vi "ODSS_Gen_Script.vi"(7 "Path":path, 8 "error in (no error)":errorcluster, 10 "Time":i32[](array[numeric]), 11 "Main Str":string) -> (0 "error out":errorcluster)   [LabVIEW 2010]
doc: "This Vi implements the routine for writing the simulation script for the next simulation step in OpenDSS.\n\nCreated by Davis Montenegro\n29-06-2017"
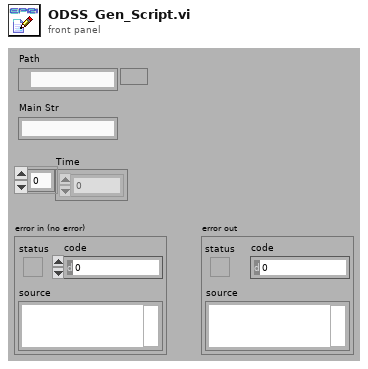
[diagram p1: front panel]
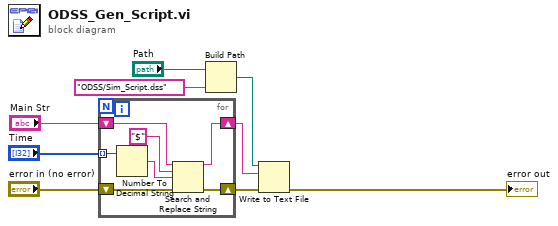
[diagram p0: block diagram]
diagram:
  n1 = for {
    shift-right: [w15] -> w7
    shift-left: "error in (no error)" -> [w14]
    tunnel: "Time" -> [w16] mode=indexing
    shift-right: [w11] -> w8
    shift-left: "Main Str" -> [w12]
    n2 = Number To Decimal String(number=w16) -> (decimal integer string=w13:string)  [unwired: 1 in]
    n3 = Search and Replace String(input string=w12, search string="$", replace string=w13, error in=w14) -> (result string=w11:string, error out=w15:errorcluster)  [unwired: 4 in, 2 out]
  }
  n4 = Build Path(base path="Path", name or relative path="ODSS/Sim_Script.dss") -> (appended path=w1:path)
  n5 = Write to Text File(file (use dialog)=w1, text=w8, error in=w7) -> (error out=→"error out":errorcluster)  [unwired: 1 in, 2 out]
